vi "Configure Triangle.vi"(0 "template configuration":refnum<class "SV Signal.lvclass">, 5 "frequency (Hz)":dbl=1000.0, 7 "amplitude":dbl=1.0, 9 "phase (deg)":dbl, 11 "error in (no error)":errorcluster, 12 "duty cycle (%)":dbl=50.0) -> (4 "signal configuration":refnum<class "SV Triangle.lvclass">, 15 "error out":errorcluster)   [LabVIEW 2017, in "SV Triangle.lvclass"]
doc: "Configures a user-defined test signal. Wire the outputs to SV Signal (waveform) VI to generate the test signal, or wire to SV Signal Property Node to configure additional parameters before wiring to the SV Signal (waveform) VI."
uses:
  <vilib>/addons/_NISVFA/_Generation/Signal Generation/SV Triangle/SV Triangle.lvclass
  C:/Program Files (x86)/National Instruments/LabVIEW 2017/vi.lib/addons/_NISVFA/_Generation/Signal Generation/SV Function/SV Function.lvclass
  C:/Program Files (x86)/National Instruments/LabVIEW 2017/vi.lib/addons/_NISVFA/_Generation/Signal Generation/SV Signal/SV Signal.lvclass
  <vilib>/addons/_NISVFA/_Generation/Signal Generation/SV Signal/SV Signal.lvclass
  <vilib>/addons/_NISVFA/_Generation/Signal Generation/SV Signal/Write Measurement Duration.vi
  <vilib>/addons/_NISVFA/_Generation/Signal Generation/SV Signal/Write Sample Rate.vi
  <vilib>/addons/_NISVFA/_Generation/Signal Generation/SV Function/SV Function.lvclass
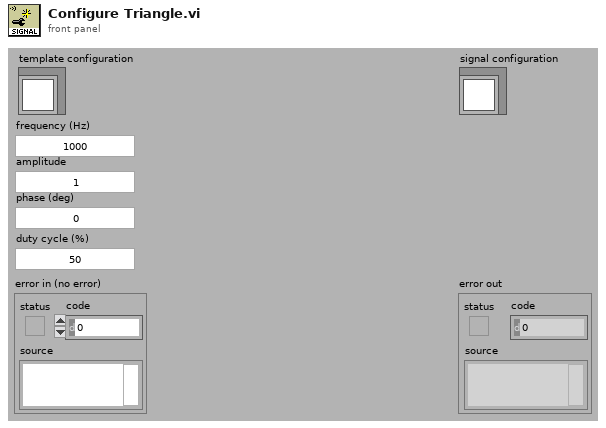
[diagram p1: front panel]
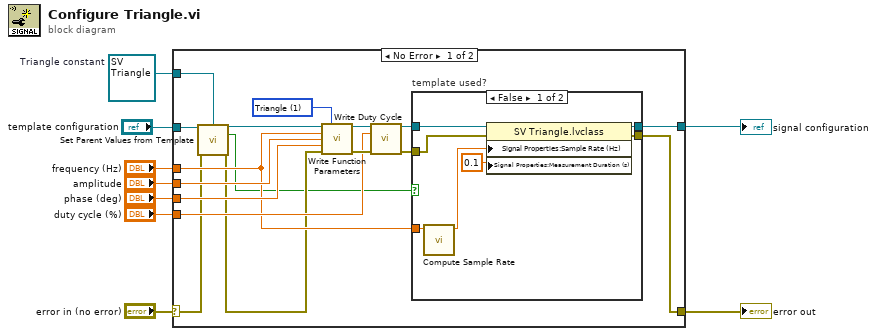
[diagram p0: block diagram]
diagram:
  w4 = refnum<class "SV Triangle.lvclass"> refnum  # Triangle constant
  n1 = case shown="No Error" "error in (no error)" {
    selector: "error in (no error)" -> [w12 w36]
    tunnel: [w16 w36] -> w8
    tunnel: [w19 w37] -> w2
    tunnel: w4 -> [w14 w37]
    tunnel: "frequency (Hz)" -> [w18 _]
    tunnel: "amplitude" -> [w26 _]
    tunnel: "phase (deg)" -> [w25 _]
    tunnel: "duty cycle (%)" -> [w21 _]
    tunnel: "template configuration" -> [w15 _]
    frame No Error {
      w24 = u16 1 items=["Sine", "Triangle", "Square", "Sawtooth"] ("function type")
      n2 = call-dynamic "Set Parent Values from Template.vi"("template configuration"=w15, "signal configuration in"=w14, "error in (no error)"=w12) -> ("signal configuration out"=w13:refnum<class "SV Triangle.lvclass">, "template used?"=w10:bool, "error out"=w11:errorcluster)  [unwired: 10 in]
      n3 = call <vilib>:"Write Function Parameters.vi"("signal configuration"=w13, "function type"=w24, "frequency (Hz)"=w18, "amplitude"=w26, "phase (deg)"=w25, "error in (no error)"=w11) -> ("signal configuration"=w23:refnum<class "SV Triangle.lvclass">, "error out"=w22:errorcluster)  [unwired: 8 in]
      n4 = call <vilib>:"Write Duty Cycle.vi"("Triangle in"=w23, "duty cycle [%]"=w21, "error in (no error)"=w22) -> ("Triangle out"=w20:refnum<class "SV Triangle.lvclass">, "error out"=w17:errorcluster)  [unwired: 11 in]
      n5 = case "template used?" shown="False" w10 {
        tunnel: w20 -> [w33 w35]
        tunnel: [w32 w35] -> w19
        tunnel: w18 -> [w31 _]
        tunnel: w17 -> [w29 w34]
        tunnel: [w28 w34] -> w16
        frame False {
          n6 = call <vilib>:"Compute Sample Rate.vi"("maximum frequency [Hz]"=w31) -> ("sample rate [Hz]"=w30:dbl)  [unwired: 10 in]
          n7 = property class="SV Triangle.lvclass"(reference=w33, error in=w29, "Signal Properties:Sample Rate (Hz)"=w30, "Signal Properties:Measurement Duration (s)"=0.1 ("Measurement Duration (s)")) -> (reference out=w32:refnum<class "SV Triangle.lvclass">, error out=w28:errorcluster)
        }
        frame True {
        }
      }
    }
    frame Error {
    }
  }
  "error out" <- w8
  "signal configuration" <- w2
